vi "getType.vi"(8 "error in (no error)":errorcluster, 11 "Scan in":refnum<class "Scan.lvclass">) -> (0 "error out":errorcluster, 2 "type":enum16{"Point", "Loop", "Scan"}(ring), 3 "Scan out":refnum<class "Scan.lvclass">)   [LabVIEW 2011, in "Tools.lvlib" / "Sequencing.lvlib" / "Scan.lvclass"]
uses:
  Scan.lvclass
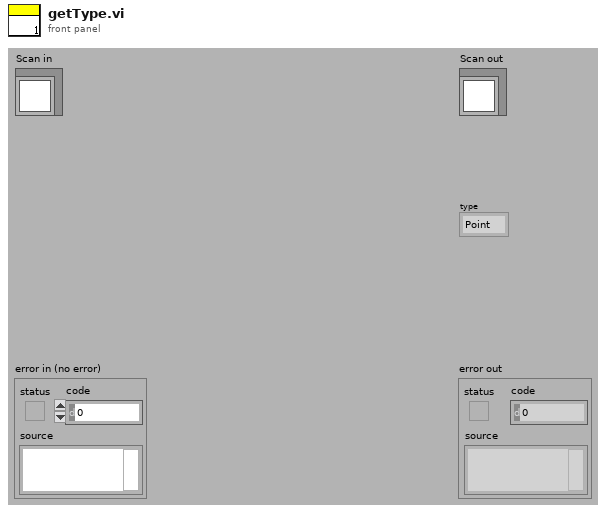
[diagram p1: front panel]
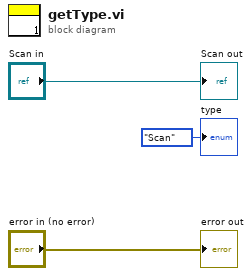
[diagram p0: block diagram]
diagram:
  "error out" <- "error in (no error)"
  "Scan out" <- "Scan in"
  "type" <- enum16{"Point", "Loop", "Scan"}."Scan" ("type")
